vi "SW_Init_Array_of_Conditions.vi"(2 "error in (no error)":T9, 3 "Array size":i32=9) -> (0 "error out":T9, 1 "Array of conditions":T1 {"Specifier(s)"."Validity criteria(s)"."Validity value" min=0.0 step=0.1 format="%.2g"; "Specifier(s)"."Value" step=1.0 format="%#.2g"})   [LabVIEW 2018, in "Common_Resources.lvlib"]
uses:
  SubVi's/Controls/CTL_Conditions_Array.ctl
  SubVi's/Controls/CTL_Conditions_Cluster.ctl
  SubVi's/Controls/CTL_Condition_type.ctl
  SubVi's/Controls/CTL_Comparison_type.ctl
  SubVi's/Controls/CTL_Validity_check_criteria.ctl
  SubVi's/Controls/CTL_Response_info.ctl
  SubVi's/Controls/CTL_Condition_response_type.ctl
  SubVi's/Controls/CTL_Reponse_port_info.ctl
  Common_Resources.lvlib
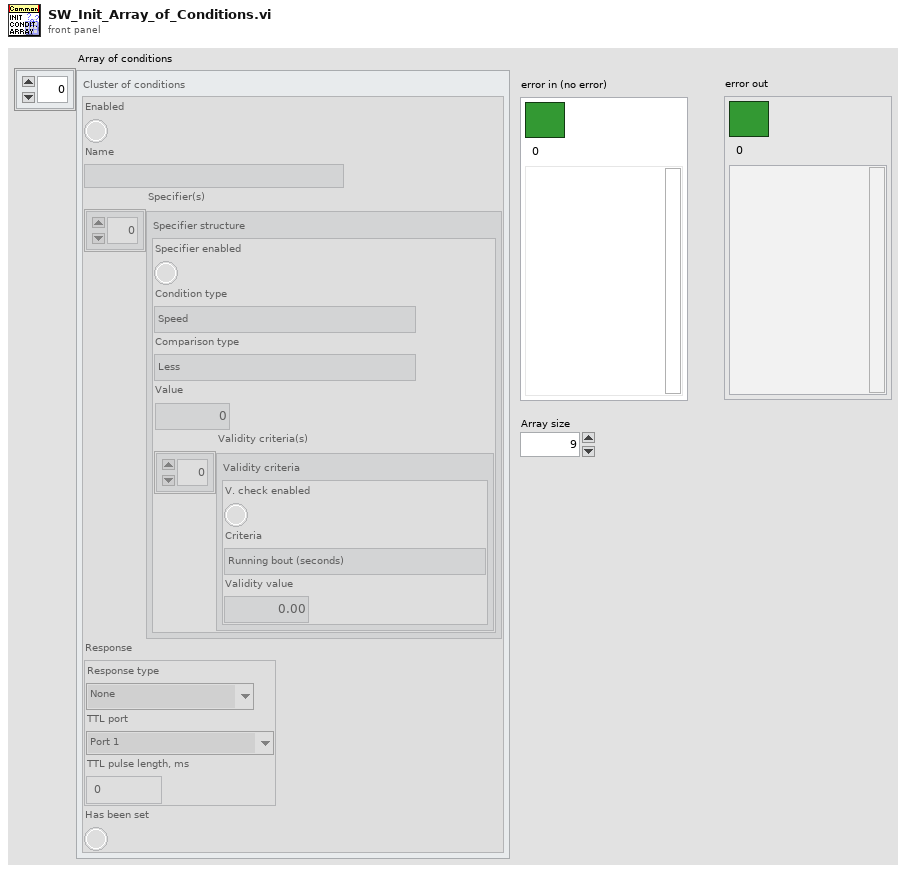
[diagram p1: front panel]
types:
  T1 = typedef "Common_Resources.lvlib/CTL_Conditions_Array.ctl" = T2[]
  T2 = typedef "Common_Resources.lvlib/CTL_Conditions_Cluster.ctl" = cluster{"Enabled":bool, "Name":string, "Specifier(s)":cluster{"Specifier enabled":bool, "Condition type":T3, "Comparison type":T4, "Value":dbl, "Validity criteria(s)":cluster{"V. check enabled":bool, "Criteria":T5, "Validity value":dbl}[]}[], "Response":T6, "Has been set":bool}
  T3 = typedef "Common_Resources.lvlib/CTL_Condition_type.ctl" = enum16{"Speed", "Zone", "Angle to wall"}
  T4 = typedef "Common_Resources.lvlib/CTL_Comparison_type.ctl" = enum16{"Less", "Less or Equal", "Equal", "Greater or Equal", "Greater", "Not Equal"}
  T5 = typedef "Common_Resources.lvlib/CTL_Validity_check_criteria.ctl" = enum16{"Running bout (seconds)", "Running bout (meters)"}
  T6 = typedef "Common_Resources.lvlib/CTL_Response_info.ctl" = cluster{"Response type":T7, "TTL port":T8, "TTL pulse length, ms":dbl}
  T7 = typedef "Common_Resources.lvlib/CTL_Condition_response_type.ctl" = enum16{"None", "Air puff", "Liquid reward", "TTL pulse", "TTL pulse (ubr)", "TTL signal"}
  T8 = typedef "Common_Resources.lvlib/CTL_Reponse_port_info.ctl" = enum16{"Port 1", "Port 2", "Port 3", "Port 4"}
  T9 = cluster{"Boolean Round":bool, "code":i32, "source":string}
  T10 = cluster{"V. check enabled":bool, "Criteria":T5, "Validity value":dbl}
  T11 = cluster{"Specifier enabled":bool, "Condition type":T3, "Limit type":T4, "Value":dbl, "Validity criteria(s)":cluster{"V. check enabled":bool, "Criteria":T5, "Validity value":dbl}[]}
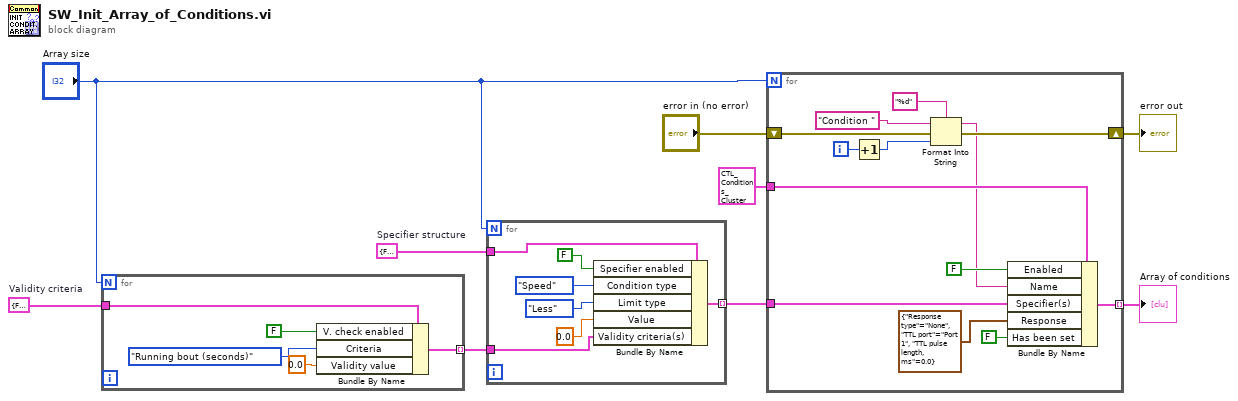
[diagram p0: block diagram]
diagram:
  w6 = T10 {"V. check enabled"=FALSE, "Criteria"=enum."Running bout (seconds)", "Validity value"=0.0}  # Validity criteria
  w9 = T11 {"Specifier enabled"=FALSE, "Condition type"=enum."Speed", "Limit type"=enum."Less", "Value"=0.0, "Validity criteria(s)"=[]}  # Specifier structure
  n1 = for {
    N: "Array size" -> [_]
    tunnel: w6 -> [w14]
    tunnel: [w10] -> w5 mode=indexing
    n2 = Bundle By Name(cluster=w14, "V. check enabled"=FALSE, "Criteria"=CTL_Validity_check_criteria."Running bout (seconds)", "Validity value"=0.0) -> (w10:T10)
  }
  n3 = for {
    N: "Array size" -> [_]
    tunnel: w9 -> [w21]
    tunnel: w5 -> [w16]
    tunnel: [w15] -> w4 mode=indexing
    n4 = Bundle By Name(cluster=w21, "Specifier enabled"=FALSE, "Condition type"=CTL_Condition_type."Speed", "Limit type"=CTL_Comparison_type."Less", "Value"=0.0, "Validity criteria(s)"=w16) -> (w15:T11)
  }
  n5 = for {
    N: "Array size" -> [_]
    tunnel: T2 {"Enabled"=FALSE, "Name"="", "Specifier(s)"=[], "Response"={"Response type"=enum."Air puff", "TTL port"=enum."Port 1", "TTL pulse length, ms"=0.0}, "Has been set"=FALSE} ("Array of conditions") -> [w34]
    tunnel: w4 -> [w32]
    tunnel: [w31] -> w3 mode=indexing
    shift-right: [w27] -> w1
    shift-left: "error in (no error)" -> [w28]
    i -> [w30]
    n6 = Increment(x=w30) -> (x+1=w24:i32)
    n7 = Format Into String(format string="%d", initial string="Condition ", error in=w28, w24) -> (resulting string=w26:string, error out=w27:errorcluster)
    n8 = Bundle By Name(cluster=w34, "Enabled"=FALSE, "Name"=w26, "Specifier(s)"=w32, "Response"=T6 {"Response type"=enum."None", "TTL port"=enum."Port 1", "TTL pulse length, ms"=0.0}, "Has been set"=FALSE) -> (w31:T2)
  }
  "error out" <- w1
  "Array of conditions" <- w3
